vi "Autonomous Mode.vi"(11 "Enum":enum16{"Init", "Run", "End"}(ring)=enum."Run") -> (3 "Autonomous":enum16{"Near", "Mid", "Far", "Disable"}(ring)=enum."Mid")   [LabVIEW 2011]
uses:
  TypeDefs/Digital Module 1.ctl
  <vilib>/Rock Robotics/SystemInterfaces/Typedef/FPGA_TypedefDigitalModule.ctl
  <vilib>/Rock Robotics/SystemInterfaces/DIO/FPGA_DIOChannel.ctl
panel:
  in  "Digital Module A":T1={"Module"=enum."Digital Module 1", "Left Enc A"=enum."DIO 1", "Left Enc B"=enum."DIO 2", "Right Enc A"=enum."DIO 3", "Right Enc B"=enum."DIO 4", "Outer Sensor"=enum."DIO 5", "Inner Sensor"=enum."DIO 6", "Upper Sensor"=enum."DIO 7", "Shooter Tachometer"=enum."DIO 8", "Unassigned"=enum."DIO 9", "Unassigned"=enum."DIO 10", "Unassigned"=enum."DIO 11", "Arm Upper Limit"=enum."DIO 12", "Arm Lower Limit"=enum."DIO 13", "1510"=enum."DIO 14"}
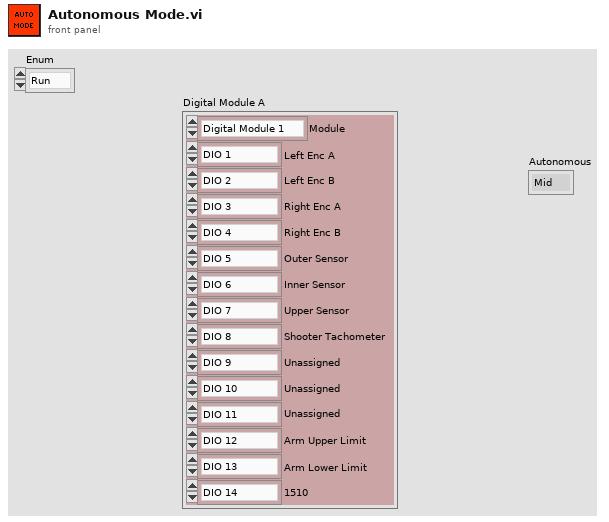
[diagram p1: front panel]
types:
  T1 = typedef "Digital Module 1.ctl" = cluster{"Module":T2, "Left Enc A":T3, "Left Enc B":T3, "Right Enc A":T3, "Right Enc B":T3, "Outer Sensor":T3, "Inner Sensor":T3, "Upper Sensor":T3, "Shooter Tachometer":T3, "Unassigned":T3, "Unassigned":T3, "Unassigned":T3, "Arm Upper Limit":T3, "Arm Lower Limit":T3, "1510":T3}
  T2 = typedef "FPGA_TypedefDigitalModule.ctl" = enum16{"Digital Module 1", "Digital Module 2"}
  T3 = typedef "FPGA_DIOChannel.ctl" = enum8{"DIO 1", "DIO 2", "DIO 3", "DIO 4", "DIO 5", "DIO 6", "DIO 7", "DIO 8", "DIO 9", "DIO 10", "DIO 11", "DIO 12", "DIO 13", "DIO 14", "Invalid"}
  T4 = typedef "WPI_DigitalInputDevRef.ctl" = cluster{"DevStatus":errorcluster, "DIO Channel":T3, "Digital Module":T2}
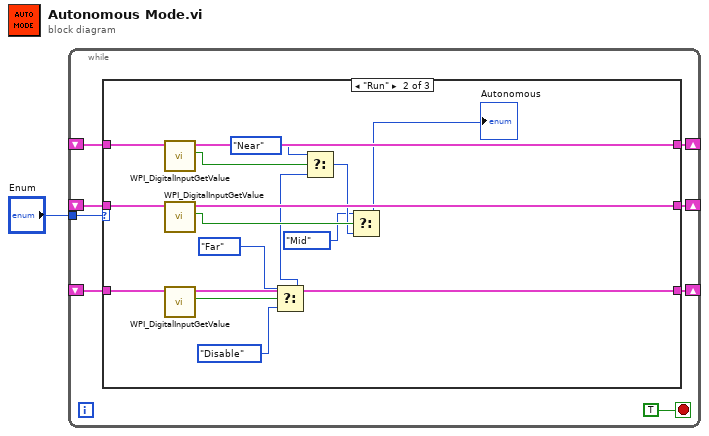
[diagram p0: block diagram]
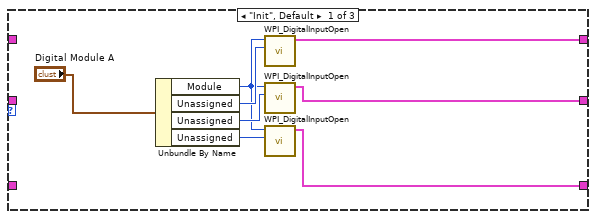
[diagram p2: hidden frame]
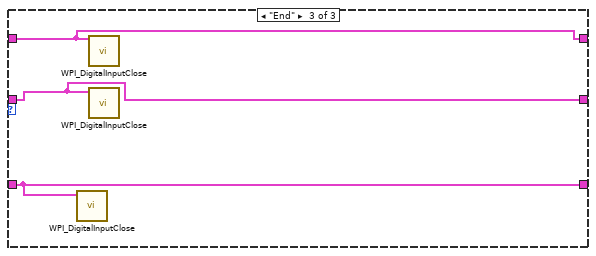
[diagram p3: hidden frame]
diagram:
  n1 = while {
    tunnel: "Enum" -> [w9]
    shift-right: [w6] -> _
    shift-left: _ -> [w2]
    shift-right: [w7] -> _
    shift-left: _ -> [w4]
    shift-right: [w8] -> _
    shift-left: _ -> [w3]
    stop <- TRUE stop-if-true
    n2 = case shown="\"Run\"" w9 {
      tunnel: [w17 w28 w34] -> w8
      tunnel: [w16 w29 w35] -> w7
      tunnel: [w15 w30 w36] -> w6
      tunnel: w4 -> [_ w33 w35]
      tunnel: w3 -> [_ w32 w34]
      tunnel: w2 -> [_ w31 w36]
      frame "Init", Default {
        n3 = Unbundle By Name("Digital Module A") -> ("Module"=w10:T2, "Unassigned"=w13:T3, "Unassigned"=w12:T3, "Unassigned"=w11:T3)
        n4 = call <vilib>:"WPI_DigitalInputOpen.vi"("DIO Channel"=w13, "Digital Module (Module 1)"=w10) -> ("DigitalInputDevRef"=w17:T4)  [unwired: 8 in, 1 out]
        n5 = call <vilib>:"WPI_DigitalInputOpen.vi"("DIO Channel"=w12, "Digital Module (Module 1)"=w10) -> ("DigitalInputDevRef"=w16:T4)  [unwired: 8 in, 1 out]
        n6 = call <vilib>:"WPI_DigitalInputOpen.vi"("DIO Channel"=w11, "Digital Module (Module 1)"=w10) -> ("DigitalInputDevRef"=w15:T4)  [unwired: 8 in, 1 out]
      }
      frame "Run" {
        n7 = call <vilib>:"WPI_DigitalInputGetValue.vi"("DigitalInputDevRef"=w32) -> ("Value"=w27:bool, "DigitalInputDevRef"=w28:T4)  [unwired: 8 in, 1 out]
        n8 = call <vilib>:"WPI_DigitalInputGetValue.vi"("DigitalInputDevRef"=w33) -> ("Value"=w26:bool, "DigitalInputDevRef"=w29:T4)  [unwired: 8 in, 1 out]
        n9 = call <vilib>:"WPI_DigitalInputGetValue.vi"("DigitalInputDevRef"=w31) -> ("Value"=w25:bool, "DigitalInputDevRef"=w30:T4)  [unwired: 8 in, 1 out]
        n10 = Select(t=enum16{"Near", "Mid", "Far", "Disable"}."Far" ("Autonomous"), s=w25, f=enum16{"Near", "Mid", "Far", "Disable"}."Disable" ("Autonomous")) -> (s? t:f=w24:enum16{"Near", "Mid", "Far", "Disable"})
        n11 = Select(t=enum16{"Near", "Mid", "Far", "Disable"}."Near" ("Autonomous"), s=w27, f=w24) -> (s? t:f=w23:enum16{"Near", "Mid", "Far", "Disable"})
        n12 = Select(t=enum16{"Near", "Mid", "Far", "Disable"}."Mid" ("Autonomous"), s=w26, f=w23) -> (s? t:f=→"Autonomous":enum16{"Near", "Mid", "Far", "Disable"})
      }
      frame "End" {
        n13 = call <vilib>:"WPI_DigitalInputClose.vi"("DigitalInputDevRef"=w36) -> ()  [unwired: 10 in, 1 out]
        n14 = call <vilib>:"WPI_DigitalInputClose.vi"("DigitalInputDevRef"=w34) -> ()  [unwired: 10 in, 1 out]
        n15 = call <vilib>:"WPI_DigitalInputClose.vi"("DigitalInputDevRef"=w35) -> ()  [unwired: 10 in, 1 out]
      }
    }
  }
